vi "Untitled 2.vi"   [LabVIEW 2019]
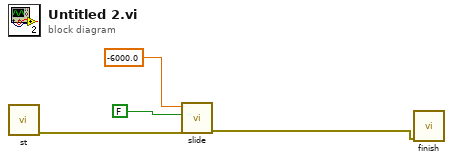
[diagram p0: block diagram]
diagram:
  n1 = call "st.vi"() -> ("Error/Flow Out"=w4:errorcluster)  [unwired: 11 in]
  n2 = call "slide.vi"("error in (no error)"=w4, "Reset Counter"=FALSE, "Numeric"=-6000.0) -> ("error out"=w3:errorcluster)  [unwired: 6 in, 2 out]
  n3 = call "finish.vi"("Error/Flow In"=w3) -> ()  [unwired: 11 in]
